vi "写入excel(幅值线性度).vi"(7 "设置":string[](array[string])=["160", "10", "0.02", "0.02", "0.1", "10", "J5", "J6"], 8 "error in (no error)":errorcluster, 9 "被测幅值":dbl format="%.2p", 10 "参考幅值":dbl format="%.2p", 11 "NI_report输入":refnum<class "NI_report.lvclass">) -> (0 "error out":errorcluster, 3 "report out":refnum<class "NI_report.lvclass">)   [LabVIEW 2015]
uses:
  <vilib>/Utility/NIReport.llb/NI_report.lvclass
  <vilib>/addons/_office/_exclsub.llb/font.ctl
  Global.vi
  <vilib>/Utility/NIReport.llb/Excel/NI_Excel.lvclass
  <vilib>/addons/_office/NI_ReportGenerationToolkit.lvlib
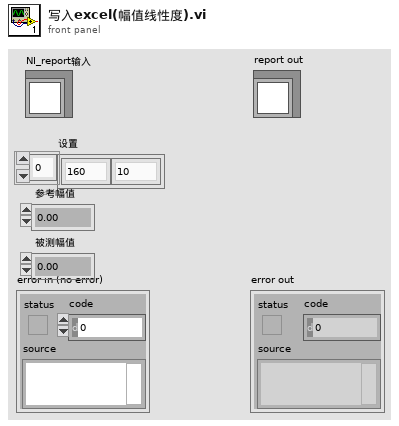
[diagram p1: front panel]
types:
  T1 = typedef "NI_ReportGenerationToolkit.lvlib/font.ctl" = cluster{"font name":string, "font size":dbl, "bold":u16, "italic":u16, "underline":u16, "strike through":u16, "font color":u32}
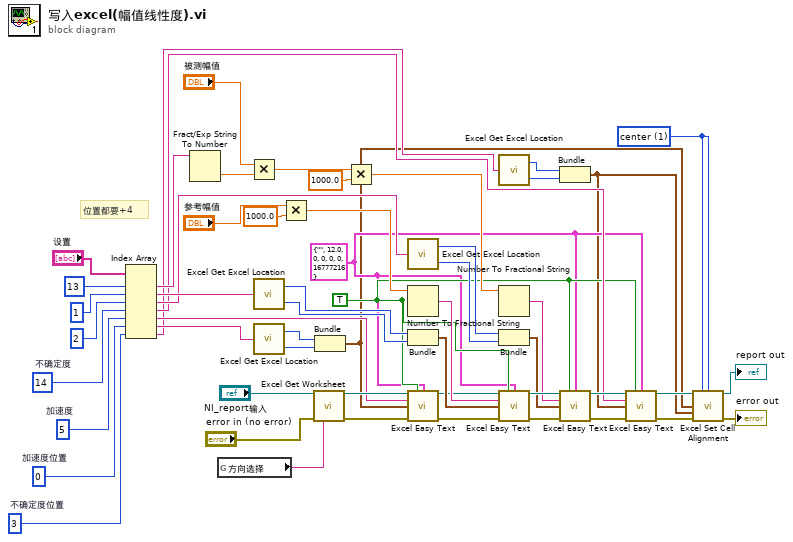
[diagram p0: block diagram]
diagram:
  w8 = 3  # 不确定度位置
  w22 = 0  # 加速度位置
  w23 = 5  # 加速度
  w24 = 14  # 不确定度
  w31 = 1 items=["top", "center", "bottom"] ("vertical alignment (top)")
  w4 = TRUE ("border? (F)")
  w3 = T1 {"font name"="", "font size"=12.0, "bold"=0, "italic"=0, "underline"=0, "strike through"=0, "font color"=16777216} ("font")
  # "位置都要+4"
  n1 = Index Array(array="设置", index #1=13 ("索引"), index #2=1 ("索引 (行)"), index #3=2 ("索引"), index #4=w24, index #5=w23, index #6=w22, index #7=w8) -> (element #1=w47:string, element #2=w44:string, element #3=w38:string, element #4=w9:string, element #5=w19:string, element #6=w18:string, element #7=w7:string)
  n2 = Fract/Exp String To Number(string=w47) -> (number=w46:dbl)  [unwired: 3 in, 1 out]
  n3 = global read "Global.vi" "方向选择"() -> (w53:string)
  n4 = Multiply(x="被测幅值", y=w46) -> (x*y=w30:dbl)
  n5 = call <vilib>:"Excel Get Excel Location.vi"("cell's name"=w44) -> ("row"=w43:i32, "column"=w42:i32)
  n6 = call <vilib>:"Excel Get Excel Location.vi"("cell's name"=w18) -> ("row"=w17:i32, "column"=w16:i32)
  n7 = Multiply(x="参考幅值", y=1000.0) -> (x*y=w25:dbl)
  n8 = call <vilib>:"Excel Get Worksheet.vi"("report in"="NI_report输入", "error in (no error)"="error in (no error)", "name (\"\")"=w53) -> ("report out"=w21:refnum<class "NI_report.lvclass">, "error out"=w20:errorcluster)  [unwired: 11 in]
  n9 = Bundle("row"=w17, "column"=w16) -> (w2:cluster{"row":i32, "column":i32})  [unwired: 1 in]
  n10 = Multiply(x=w30, y=1000.0) -> (x*y=w28:dbl)
  n11 = call <vilib>:"Excel Get Excel Location.vi"("cell's name"=w38) -> ("row"=w37:i32, "column"=w36:i32)
  n12 = Number To Fractional String(number=w25) -> (F-format string=w45:string)  [unwired: 3 in]
  n13 = Bundle("row"=w43, "column"=w42) -> (w33:cluster{"row":i32, "column":i32})  [unwired: 1 in]
  n14 = call <vilib>:"Excel Easy Text.vi"("report in"=w21, "border? (F)"=w4, "font"=w3, "text"=w19, "start (-1, -1)"=w2, "error in (no error)"=w20) -> ("report out"=w15:refnum<class "NI_report.lvclass">, "error out"=w14:errorcluster)  [unwired: 5 in, 3 out]
  n15 = call <vilib>:"Excel Get Excel Location.vi"("cell's name"=w7) -> ("row"=w6:i32, "column"=w5:i32)
  n16 = Number To Fractional String(number=w28) -> (F-format string=w39:string)  [unwired: 3 in]
  n17 = Bundle("row"=w37, "column"=w36) -> (w32:cluster{"row":i32, "column":i32})  [unwired: 1 in]
  n18 = call <vilib>:"Excel Easy Text.vi"("report in"=w15, "border? (F)"=w4, "font"=w3, "text"=w45, "start (-1, -1)"=w33, "error in (no error)"=w14) -> ("report out"=w41:refnum<class "NI_report.lvclass">, "error out"=w40:errorcluster)  [unwired: 5 in, 3 out]
  n19 = Bundle("row"=w6, "column"=w5) -> (w1:cluster{"row":i32, "column":i32})  [unwired: 1 in]
  n20 = call <vilib>:"Excel Easy Text.vi"("report in"=w41, "border? (F)"=w4, "font"=w3, "text"=w39, "start (-1, -1)"=w32, "error in (no error)"=w40) -> ("report out"=w13:refnum<class "NI_report.lvclass">, "error out"=w12:errorcluster)  [unwired: 5 in, 3 out]
  n21 = call <vilib>:"Excel Easy Text.vi"("report in"=w13, "border? (F)"=w4, "font"=w3, "text"=w9, "start (-1, -1)"=w1, "error in (no error)"=w12) -> ("report out"=w11:refnum<class "NI_report.lvclass">, "error out"=w10:errorcluster)  [unwired: 5 in, 3 out]
  n22 = call <vilib>:"Excel Set Cell Alignment.vi"("report in"=w11, "vertical alignment (top)"=w31, "horizontal alignment (left)"=w31, "start (-1, -1)"=w2, "end (-1, -1)"=w1, "error in (no error)"=w10) -> ("report out"=→"report out":refnum<class "NI_report.lvclass">, "error out"=→"error out":errorcluster)  [unwired: 8 in]
